vi "dfd_IPGen_Global.vi"() -> ()   [LabVIEW 2017, in "NI_DigFilter_IPGenerator.lvlib"]
uses:
  <vilib>/addons/Digital Filter Design/NI_DigFilter_IPGenerator.lvlib
panel:
  in  "FPGA clock rate":dbl=40000000.0 format="%#_6p"
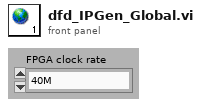
[diagram p1: front panel]
diagram:
